vi "Buffer.vi"(7 "Functions":T1, 8 "error in (no error)":errorcluster, 10 "Config in":refnum<class "Carya Config.lvclass">, 11 "Carya Config (Buffer) in":refnum<class "CConfig By Ref Buffer.lvclass">) -> (0 "error out":errorcluster, 1 "queue out":refnum<queue>, 2 "Config out":refnum<class "Carya Config.lvclass">, 3 "Carya Config (Buffer) out":refnum<class "CConfig By Ref Buffer.lvclass">, 4 "Wait\\Check":bool=TRUE)   [LabVIEW 2013, in "CConfig By Ref Buffer.lvclass"]
doc: "Copyright 2018, Carya Automatisering, Wiebe Walstra."
uses:
  CConfig By Ref Buffer.lvclass
  Buffer Functions.ctl
  Carya Config.lvclass
  CConfig By Ref Buffer.lvclass/CConfig By Ref Buffer.ctl
  <vilib>/Utility/error.llb/Error Cluster From Error Code.vi
  <vilib>/ErrorRing/Error Ring.xnode
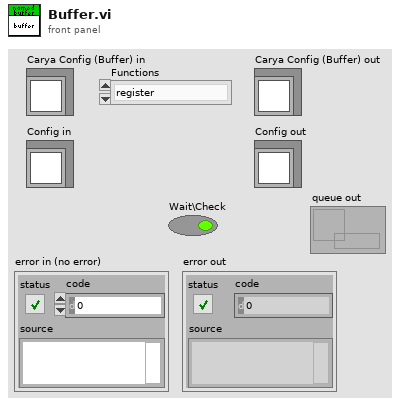
[diagram p1: front panel]
types:
  T1 = typedef "CConfig By Ref Buffer.lvclass/Buffer Functions.ctl" = enum16{"register", "get and lock", "set and unlock", "unlock", "unregister", "check"}
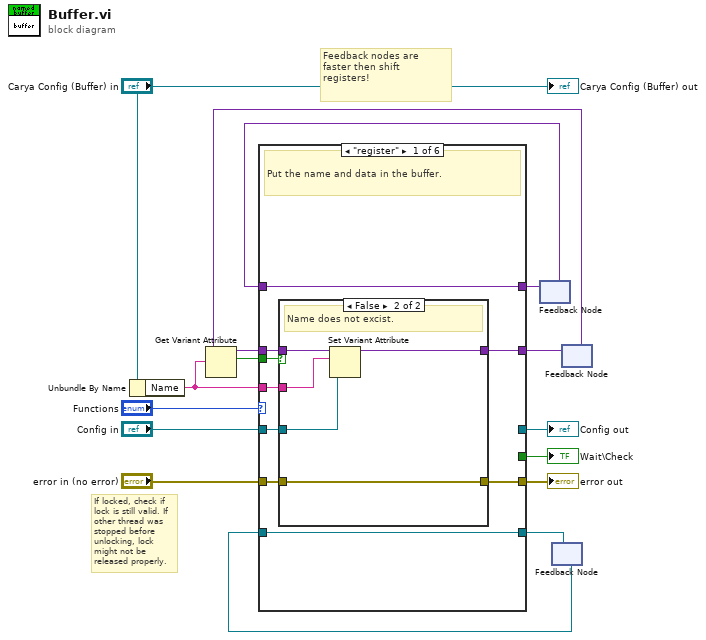
[diagram p0: block diagram]
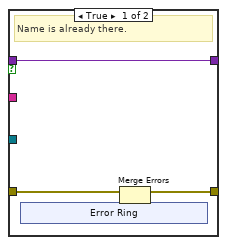
[diagram p2: hidden frame]
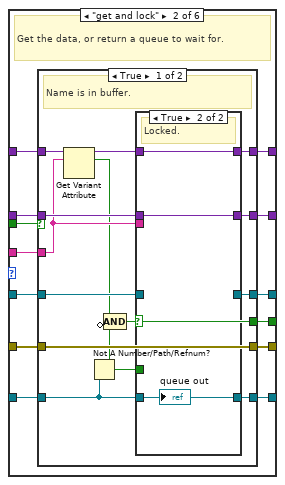
[diagram p3: hidden frame]
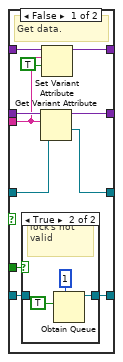
[diagram p4: hidden frame]
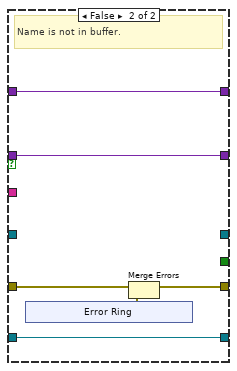
[diagram p6: hidden frame]
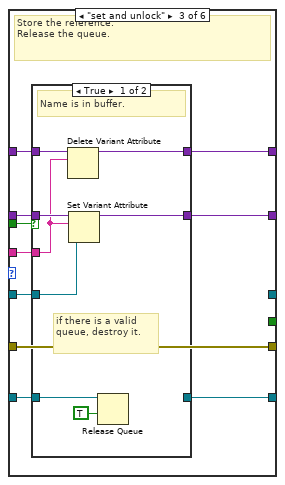
[diagram p7: hidden frame]
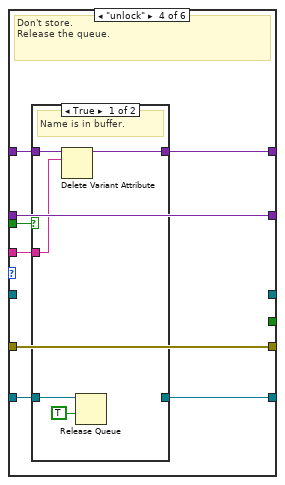
[diagram p9: hidden frame]
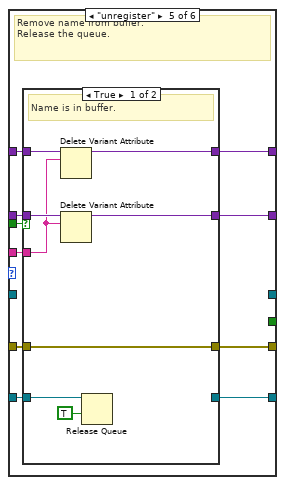
[diagram p11: hidden frame]
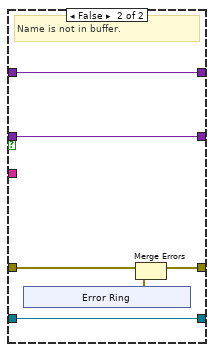
[diagram p12: hidden frame]
diagram:
  # "Feedback nodes are faster then shift registers!"
  # "If locked, check if lock is still valid. If other thread was stopped before unlocking, lock might not be released properly."
  n1 = Unbundle By Name("Carya Config (Buffer) in") -> ("Name"=w10:string)
  n2 = feedback #1() -> (w7:variant)  [unwired: 1 in]
  n3 = feedback #2() -> (w3:refnum<queue>)  [unwired: 1 in]
  n4 = feedback #3() -> (w5:variant)  [unwired: 1 in]
  n5 = Get Variant Attribute(Variant=w5, name=w10) -> (duplicate Variant=w1:variant, found=w2:bool)  [unwired: 2 in, 2 out]
  n6 = case shown="\"register\"" "Functions" {
    tunnel: "error in (no error)" -> [w25 w51 w105 w124 w141 w165]
    tunnel: [w24 w52 w105 w124 w140 w165] -> w15
    tunnel: w10 -> [w23 w48 w104 w123 w139 _]
    tunnel: [_ w50 _ _ _ _] -> w14
    tunnel: [_ w49 _ _ _ w164] -> w13
    tunnel: "Config in" -> [w22 w44 w96 _ _ _]
    tunnel: w2 -> [w21 w47 w103 w122 w136 w164]
    tunnel: w1 -> [w20 w46 w102 w121 w138 w163]
    tunnel: [w19 w45 w101 w121 w137 w163] -> w6
    tunnel: w3 -> [w17 w40 w98 w118 w135 w161]
    tunnel: w7 -> [w18 w43 w100 w120 w134 w162]
    tunnel: [w18 w42 w99 w119 w133 w162] -> w8
    tunnel: [w17 w41 w97 w117 w132 w161] -> w4
    frame "register" {
      # "Put the name and data in the buffer."
      n7 = case shown="False" w21 {
        tunnel: w25 -> [w29 w39]
        tunnel: [w28 w39] -> w24
        tunnel: w23 -> [_ w37]
        tunnel: w22 -> [_ w35]
        tunnel: w20 -> [w26 w38]
        tunnel: [w26 w36] -> w19
        frame True {
          # "Name is already there."
          n8 = xnode "Error Ring"() -> ("error out"=w27:errorcluster)
          n9 = Merge Errors(w29, w27) -> (w28:errorcluster)
        }
        frame False {
          # "Name does not excist."
          n10 = Set Variant Attribute(Variant=w38, name=w37, value=w35) -> (Variant out=w36:variant)  [unwired: 1 in, 2 out]
        }
      }
    }
    frame "get and lock" {
      # "Get the data, or return a queue to wait for."
      n11 = case shown="True" w47 {
        tunnel: [w66 w88] -> w52
        tunnel: w51 -> [w66 w89]
        tunnel: [w65 _] -> w50
        tunnel: [w53 _] -> w49
        tunnel: w48 -> [w60 _]
        tunnel: w46 -> [w64 w87]
        tunnel: [w63 w87] -> w45
        tunnel: w44 -> [w62 _]
        tunnel: w43 -> [w61 w86]
        tunnel: [w59 w86] -> w42
        tunnel: [w57 w85] -> w41
        tunnel: w40 -> [w56 w85]
        frame True {
          # "Name is in buffer."
          n12 = Get Variant Attribute(Variant=w61, name=w60) -> (duplicate Variant=w58:variant, found=w55:bool)  [unwired: 2 in, 2 out]
          n13 = Not A Number/Path/Refnum?(number/path/refnum=w56) -> (NaN/Path/Refnum?=w54:bool)
          n14 = Compound Arithmetic op=AND(w55, invert w54) -> (w53:bool)
          n15 = case shown="True" w53 {
            tunnel: [w75 _] -> w65
            tunnel: w64 -> [w77 w84]
            tunnel: [w76 w84] -> w63
            tunnel: w60 -> [w71 _]
            tunnel: w62 -> [w74 _]
            tunnel: [w72 w83] -> w59
            tunnel: w58 -> [w73 w83]
            tunnel: w56 -> [w69 w82]
            tunnel: [w68 w82] -> w57
            tunnel: w54 -> [w67 _]
            frame False {
              # "Get data."
              n16 = case shown="True" w67 {
                tunnel: w69 -> [w78 _]
                tunnel: [w78 w79] -> w68
                frame False {
                  # "Lock is valid."
                }
                frame True {
                  # "lock's not valid"
                  n17 = Obtain Queue(max queue size (-1, unlimited)=1, element data type=TRUE) -> (queue out=w79:refnum<queue>)  [unwired: 3 in, 2 out]
                }
              }
              n18 = Get Variant Attribute(Variant=w77, name=w71, default value (empty Variant)=w74) -> (duplicate Variant=w76:variant, value=w75:refnum<class "Carya Config.lvclass">)  [unwired: 1 in, 2 out]
              n19 = Set Variant Attribute(Variant=w73, name=w71, value=TRUE) -> (Variant out=w72:variant)  [unwired: 1 in, 2 out]
            }
            frame True {
              # "Locked."
              "queue out" <- w82
            }
          }
        }
        frame False {
          # "Name is not in buffer."
          n20 = xnode "Error Ring"() -> ("error out"=w90:errorcluster)
          n21 = Merge Errors(w89, w90) -> (w88:errorcluster)
        }
      }
    }
    frame "set and unlock" {
      # "Store the reference.\nRelease the queue."
      n22 = case shown="True" w103 {
        tunnel: w96 -> [w106 _]
        tunnel: w104 -> [w109 _]
        tunnel: w102 -> [w113 w116]
        tunnel: [w112 w116] -> w101
        tunnel: w100 -> [w111 w115]
        tunnel: [w110 w115] -> w99
        tunnel: w98 -> [w108 w114]
        tunnel: [_ w114] -> w97
        frame True {
          # "if there is a valid queue, destroy it."
          # "Name is in buffer."
          n23 = Delete Variant Attribute(6:w109, 7:w111) -> (3:w110:variant)  [unwired: 1 in, 2 out]
          n24 = Set Variant Attribute(Variant=w113, name=w109, value=w106) -> (Variant out=w112:variant)  [unwired: 1 in, 2 out]
          n25 = Release Queue(queue=w108, force destroy? (F)=TRUE) -> ()  [unwired: 1 in, 3 out]
        }
        frame False {
          # "Name is not in buffer."
        }
      }
    }
    frame "unlock" {
      # "Don't store.\nRelease the queue."
      n26 = case shown="True" w122 {
        tunnel: w123 -> [w127 _]
        tunnel: w120 -> [w129 w131]
        tunnel: [w128 w131] -> w119
        tunnel: w118 -> [w126 w130]
        tunnel: [_ w130] -> w117
        frame True {
          # "Name is in buffer."
          n27 = Delete Variant Attribute(6:w127, 7:w129) -> (3:w128:variant)  [unwired: 1 in, 2 out]
          n28 = Release Queue(queue=w126, force destroy? (F)=TRUE) -> ()  [unwired: 1 in, 3 out]
        }
        frame False {
          # "Name is not in buffer."
        }
      }
    }
    frame "unregister" {
      # "Remove name from buffer.\nRelease the queue."
      n29 = case shown="True" w136 {
        tunnel: w141 -> [w149 w155]
        tunnel: [w149 w154] -> w140
        tunnel: w139 -> [w144 _]
        tunnel: w138 -> [w148 w152]
        tunnel: [w147 w152] -> w137
        tunnel: w135 -> [w143 w150]
        tunnel: w134 -> [w146 w151]
        tunnel: [w145 w151] -> w133
        tunnel: [_ w150] -> w132
        frame True {
          # "Name is in buffer."
          n30 = Delete Variant Attribute(6:w144, 7:w146) -> (3:w145:variant)  [unwired: 1 in, 2 out]
          n31 = Delete Variant Attribute(6:w144, 7:w148) -> (3:w147:variant)  [unwired: 1 in, 2 out]
          n32 = Release Queue(queue=w143, force destroy? (F)=TRUE) -> ()  [unwired: 1 in, 3 out]
        }
        frame False {
          # "Name is not in buffer."
          n33 = xnode "Error Ring"() -> ("error out"=w153:errorcluster)
          n34 = Merge Errors(w155, w153) -> (w154:errorcluster)
        }
      }
    }
    frame "check" {
      # "Check if name is in buffer."
    }
  }
  "error out" <- w15
  "Config out" <- w14
  "Wait\\Check" <- w13
  n35 = feedback-in #1(w8) -> ()
  n36 = feedback-in #2(w4) -> ()
  n37 = feedback-in #3(w6) -> ()
  "Carya Config (Buffer) out" <- "Carya Config (Buffer) in"
